vi "testing extract_1.vi"() -> ()   [LabVIEW 2011]
uses:
  Program Files (x86)/National Instruments/Biomedical Startup Kit Source Code/Shared/File IO/SubVI/biosignal_fileload_settings.ctl
  <vilib>/Platform/TimedLoop/XDataNode/timing_clust.ctl
  <vilib>/Platform/TimedLoop/XDataNode/nitl_modes.ctl
  <vilib>/Platform/TimedLoop/XDataNode/wakeup.ctl
  <vilib>/Platform/TimedLoop/XDataNode/XDataNode.xnode
  <vilib>/Platform/TimedLoop/XDataNode/XDNodeRunTimeDep.lvlib
panel:
  out "Tp":i32
  out "iso level":dbl
  out "beat end":i32
  out "qrs offset":i32
  out "qrs onset":i32
  out "R":i32
  out "p offset":i32
  out "beat start":i32
  out "t onset":i32
  in  "dt":dbl=0.005
  out "Numeric":dbl
  in  "millisecond multiple 3":u32=1000
  out "heart rate":i32
  in  "threshold factor":dbl=0.3125
  out "size(s)":i32
  out "QRS detected? 2":bool
  out "detected QRS peak 2":dbl[](array[numeric])
  out "detected QRS time 2":dbl[](array[numeric]) format="%<%H:%M:%S%3u>t"
  in  "millisecond multiple 2":u32=1000
  out "Waveform Out":waveform(dbl)(graph)
  in  "stop":bool
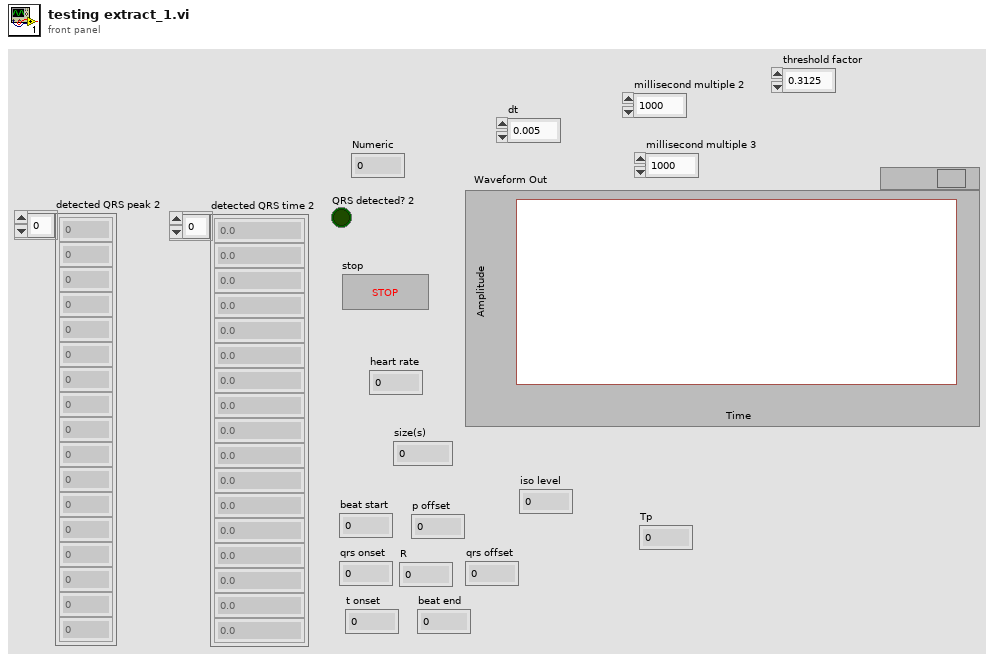
[diagram p1: front panel]
types:
  T1 = typedef "biosignal_fileload_settings.ctl" = cluster{"file path":path, "format":string, "channel name":string, "start (sample)":u32, "block size (sample)":u32, "init? (T)":bool, "group name":string, "cluster / waveform?":bool, "out ann?":bool, "length (sample)":u32, "sample rate":dbl, "unit string":string}
  T2 = typedef "XDNodeRunTimeDep.lvlib/timing_clust.ctl" = cluster{"Expected End [f-1]":u64, "Actual End [f-1]":u64, "Finished Late? [f-1]":bool, "Expected End [i-1]":u64, "Actual End [i-1]":u64, "Finished Late? [i-1]":bool, "Expected Start [i]":u64, "Actual Start [i]":u64, "Expected Start [f]":u64, "Actual Start [f]":u64, "Source Name":string, "Structure Name":string, "Period":i64, "Deadline":i64, "Offset":i64, "Start":i64, "Priority":i32, "Timeout":i32, "Mode":T3, "Wakeup Reason":T4, "Error":errorcluster, "Source Type":string, "Secondary Source Type":string, "Global End Time":u64, "Global Start Time":u64, "Frame Duration":u64, "Iteration Duration":u64, "Assigned CPU":i32, "I/O Scan Engine Mode":u32}
  T3 = typedef "XDNodeRunTimeDep.lvlib/nitl_modes.ctl" = enum32{"No Change", "Process missed periods, maintain original phase", "Discard missed periods, maintain original phase", "Process missed periods, ignore original phase", "Discard missed periods, ignore original phase"}
  T4 = typedef "XDNodeRunTimeDep.lvlib/wakeup.ctl" = enum32{"Normal", "Aborted", "Asynchronous wakeup", "Timing source error", "Timed loop error", "Timeout"}
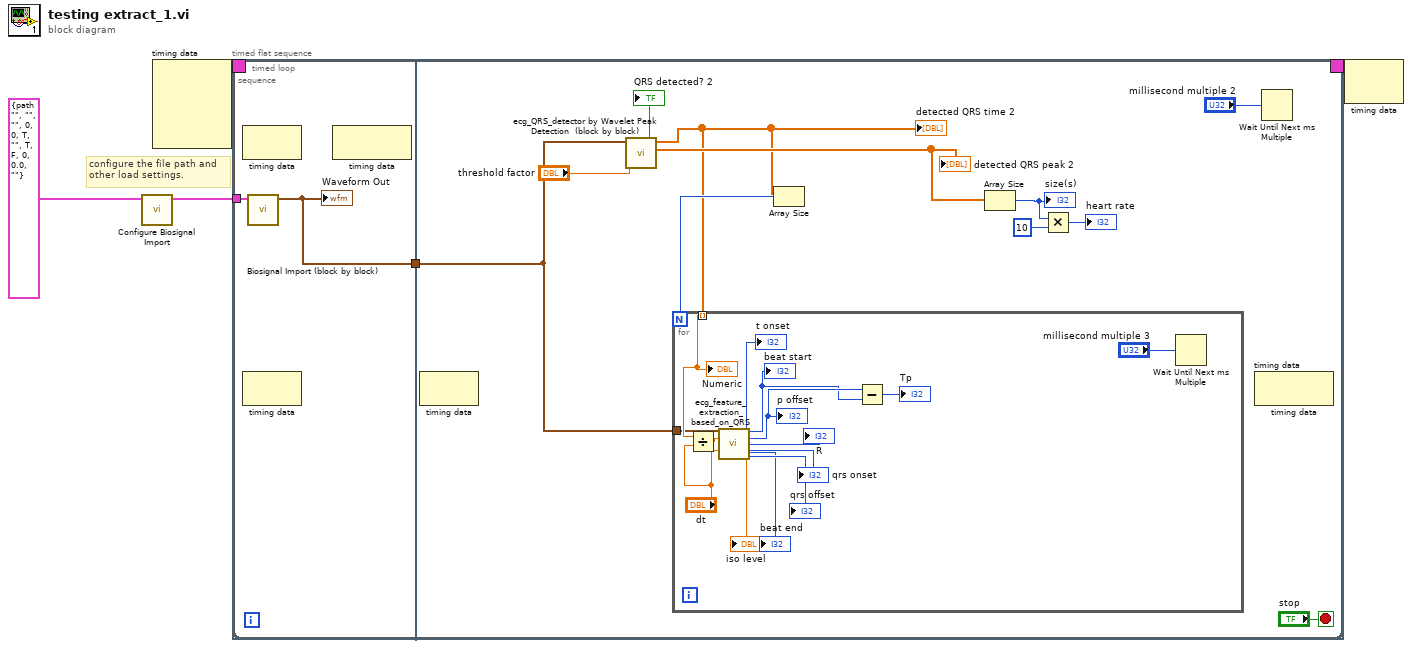
[diagram p0: block diagram]
diagram:
  # "configure the file path and\nother load settings."
  n1 = call "Configure Biosignal Import.vi"("import settings"=T1 {"file path"=path "", "format"="", "channel name"="", "start (sample)"=0, "block size (sample)"=0, "init? (T)"=TRUE, "group name"="", "cluster / waveform?"=TRUE, "out ann?"=FALSE, "length (sample)"=0, "sample rate"=0.0, "unit string"=""}) -> ("import settings out"=w3:T1)  [unwired: 9 out]
  n2 = node-c288() -> (w2:T2)  [unwired: 4 in]
  n3 = timed-loop {
    tunnel: w3 -> [w5]
    timing: w2 -> [_]
    timing-out: [_] -> w1
    stop <- "stop" stop-if-true
    n4 = timed-sequence {
      timing: _ -> [_]
      timing-out: _ -> [_]
      tunnel: w5 -> [w7]
      n5 = timed-flat-sequence {
        tunnel: w7 -> [w9]
        tunnel: [w8] -> w6
        tunnel: w6 -> [w12]
        frame #0 {
          n6 = node-c288() -> ()  [unwired: 1 in, 1 out]
          n7 = call "Biosignal Import (block by block).vi"("import settings"=w9) -> ("biosignal waveform"=w8:waveform(dbl))  [unwired: 6 in, 4 out]
          "Waveform Out" <- w8
          n8 = node-c288() -> ()  [unwired: 1 in, 1 out]
        }
        frame #1 {
          n9 = node-c288() -> ()  [unwired: 1 in, 1 out]
          n10 = call "ecg_QRS_detector by Wavelet Peak Detection  (block by block).vi"("threshold factor"="threshold factor", "ECG in"=w12) -> ("QRS detected?"=→"QRS detected? 2":bool, "detected QRS peak"=w19:dbl[], "detected QRS time"=w13:dbl[])  [unwired: 7 in]
          "detected QRS time 2" <- w13
          "detected QRS peak 2" <- w19
          n11 = Array Size(array=w13) -> (size(s)=w14:i32)
          n12 = for {
            N: w14 -> [_]
            tunnel: w13 -> [w34] mode=indexing
            tunnel: w12 -> [w26]
            n13 = Divide(x=w34, y="dt") -> (x/y=w35:dbl)
            n14 = call "ecg_feature_extraction_based_on_QRS.vi"("ECG (1s)"=w26, "R pos (index)"=w35, "dt"="dt") -> ("t onset"=→"t onset":i32, "beat start"=w24:i32, "p offset"=w25:i32, "R"=→"R":i32, "qrs onset"=→"qrs onset":i32, "iso level"=→"iso level":dbl, "beat end"=→"beat end":i32, "qrs offset"=→"qrs offset":i32)  [unwired: 3 in, 2 out]
            "beat start" <- w24
            "p offset" <- w25
            n15 = Subtract(x=w25, y=w24) -> (x-y=→"Tp":i32)
            n16 = Wait Until Next ms Multiple(millisecond multiple="millisecond multiple 3") -> ()  [unwired: 1 out]
            "Numeric" <- w34
          }
          n17 = Array Size(array=w19) -> (size(s)=w17:i32)
          "size(s)" <- w17
          n18 = Multiply(x=w17, y=10) -> (x*y=→"heart rate":i32)
          n19 = node-c288() -> ()  [unwired: 1 in, 1 out]
          n20 = Wait Until Next ms Multiple(millisecond multiple="millisecond multiple 2") -> ()  [unwired: 1 out]
        }
      }
    }
    n21 = node-c288() -> ()  [unwired: 1 in, 1 out]
    n22 = node-c288() -> ()  [unwired: 1 in, 1 out]
  }
  n23 = node-c288(w1) -> ()  [unwired: 1 out]
